vi "SwapInstanceVIUnusedName2 43.vi"(6 "Bindata & descr in":T1, 7 "type":dbl, 8 "error in (no error)":errorcluster, 9 "dims":u8=3 min=1 max=3, 11 "kwarg_name":string="testarg") -> (0 "error out":errorcluster, 1 "Array 3D":dbl[][][](array[numeric]) format="%.2f", 2 "Array 2D":dbl[][](array[numeric]) format="%.2f", 3 "Array 1D":dbl[](array[numeric]) format="%.2f", 4 "Bindata & descr out":T1, 5 "bindata":u8[](array[numeric]))   [LabVIEW 2018]
uses:
  Bindata&description.ctl
  Bindata description.ctl
  212a36f8-8f57-49c9-9677-432581b68510.vi
  69652d2b-db18-4aab-bd2f-35078bef0426.vi
  4772bca8-5d3a-4f2a-8bbf-c07de0696f94.vi
  7139aa7f-98bf-4369-975b-4bd5deaf00da.vi
  69652d2b-db18-4aab-bd2f-35078bef0426.vi/dfcf8de0-7860-4713-ab77-0e8f714dde10.vi
  4772bca8-5d3a-4f2a-8bbf-c07de0696f94.vi/e532232b-f4b6-4bbd-a5e7-664623875ae8.vi
  7139aa7f-98bf-4369-975b-4bd5deaf00da.vi/7a16f954-d622-4be0-bb4d-b4bfb8ef0f01.vi
  69652d2b-db18-4aab-bd2f-35078bef0426.vi/dfcf8de0-7860-4713-ab77-0e8f714dde10.vi/9577cbac-8520-44d1-a8fc-fc5a580fd613.vi
  4772bca8-5d3a-4f2a-8bbf-c07de0696f94.vi/e532232b-f4b6-4bbd-a5e7-664623875ae8.vi/9588a387-4c4f-45f1-904b-84c07455829b.vi
  7139aa7f-98bf-4369-975b-4bd5deaf00da.vi/7a16f954-d622-4be0-bb4d-b4bfb8ef0f01.vi/9c88b2f3-976e-4a83-96e4-93271b3fbf6a.vi
  69652d2b-db18-4aab-bd2f-35078bef0426.vi/dfcf8de0-7860-4713-ab77-0e8f714dde10.vi/9577cbac-8520-44d1-a8fc-fc5a580fd613.vi/fbec7817-6f14-44c2-b008-b20ff5437b8a.vi
  4772bca8-5d3a-4f2a-8bbf-c07de0696f94.vi/e532232b-f4b6-4bbd-a5e7-664623875ae8.vi/9588a387-4c4f-45f1-904b-84c07455829b.vi/4f801452-6626-4e48-a8e0-47d2bc6ca629.vi
  7139aa7f-98bf-4369-975b-4bd5deaf00da.vi/7a16f954-d622-4be0-bb4d-b4bfb8ef0f01.vi/9c88b2f3-976e-4a83-96e4-93271b3fbf6a.vi/05c0184e-e222-4767-93e3-5fbdd5e0ae8f.vi
  check ID validity.vi
  LV-Julia_ZMQ-Roundtrip_lib.lvlib
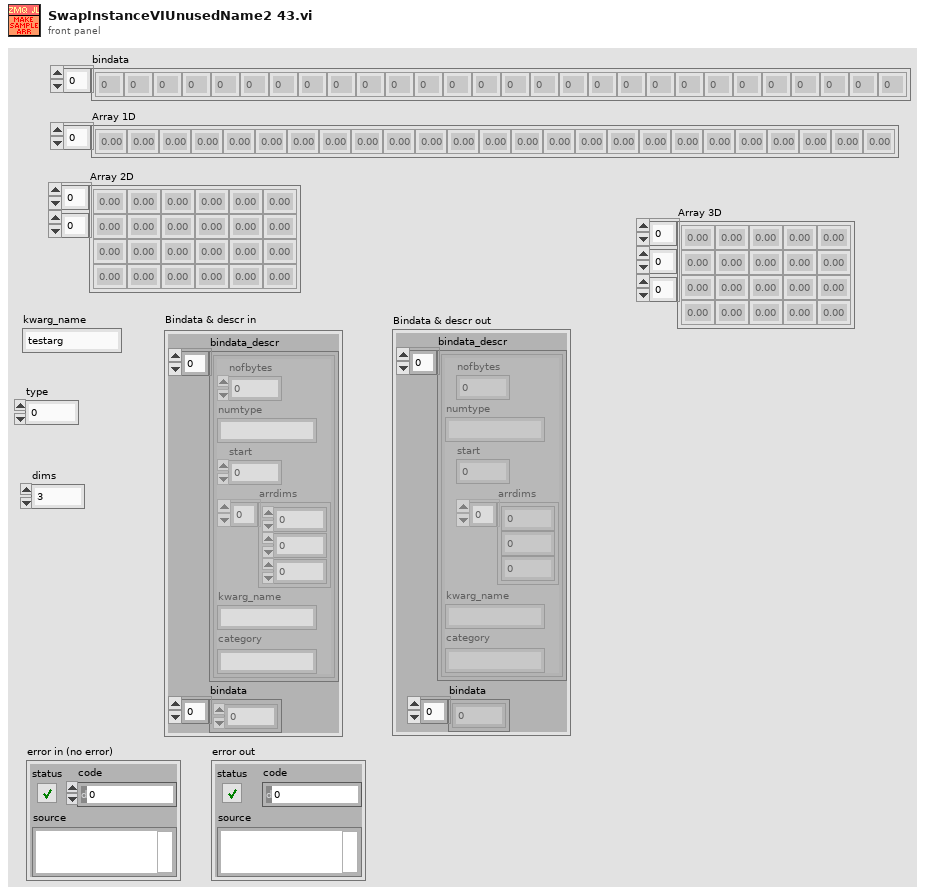
[diagram p1: front panel]
types:
  T1 = typedef "Bindata&description.ctl" = cluster{"bindata_descr":T2[], "bindata":u8[]}
  T2 = typedef "LV-Julia_ZMQ-Roundtrip_lib.lvlib/Bindata description.ctl" = cluster{"nofbytes":i32, "numtype":string, "start":i32, "arrdims":i32[], "kwarg_name":string, "category":string}
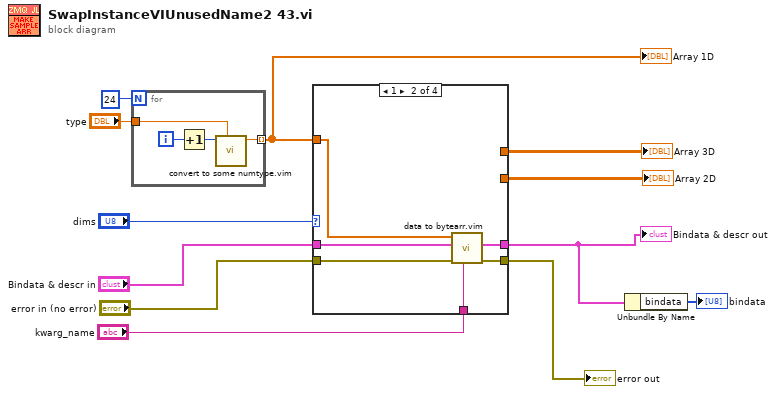
[diagram p0: block diagram]
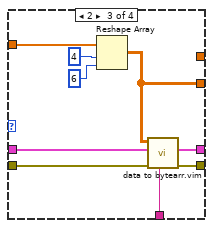
[diagram p3: hidden frame]
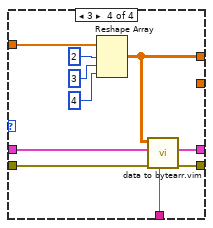
[diagram p4: hidden frame]
diagram:
  n1 = for {
    N: 24 -> [_]
    tunnel: [w14] -> w11 mode=indexing
    tunnel: "type" -> [w13]
    i -> [w16]
    n2 = Increment(x=w16) -> (x+1=w15:i32)
    n3 = call "convert to some numtype.vim"("type"=w13, "Numeric in"=w15) -> ("Numeric out"=w14:dbl)  [unwired: 9 in]
  }
  "Array 1D" <- w11
  n4 = case shown="1" "dims" {
    tunnel: [_ _ _ w42] -> w12
    tunnel: w11 -> [_ w23 w30 w38]
    tunnel: "kwarg_name" -> [_ w22 w29 w37]
    tunnel: "error in (no error)" -> [w17 w21 w28 w36]
    tunnel: [w17 w20 w27 w35] -> w5
    tunnel: [_ w19 w26 w34] -> w2
    tunnel: [_ _ w25 _] -> w4
    tunnel: "Bindata & descr in" -> [_ w18 w24 w33]
    frame 0, Default {
    }
    frame 1 {
      n5 = call "data to bytearr.vim"("kwarg_name"=w22, "error in (no error)"=w21, "Bindata & descr in"=w18, "data in"=w23) -> ("error out"=w20:errorcluster, "Bindata & descr out"=w19:T1)  [unwired: 5 in, 1 out]
    }
    frame 2 {
      n6 = Reshape Array(w30, 4 ("dimension size"), 6 ("dimension size")) -> (w25:dbl[][])
      n7 = call "data to bytearr.vim"("kwarg_name"=w29, "error in (no error)"=w28, "Bindata & descr in"=w24, "data in"=w25) -> ("error out"=w27:errorcluster, "Bindata & descr out"=w26:T1)  [unwired: 5 in, 1 out]
    }
    frame 3 {
      n8 = Reshape Array(w38, 2 ("dimension size"), 3 ("dimension size"), 4 ("dimension size")) -> (w42:dbl[][][])
      n9 = call "data to bytearr.vim"("kwarg_name"=w37, "error in (no error)"=w36, "Bindata & descr in"=w33, "data in"=w42) -> ("error out"=w35:errorcluster, "Bindata & descr out"=w34:T1)  [unwired: 5 in, 1 out]
    }
  }
  "Array 3D" <- w12
  "Bindata & descr out" <- w2
  "error out" <- w5
  "Array 2D" <- w4
  n10 = Unbundle By Name(w2) -> ("bindata"=→"bindata":u8[])
